vi "solar_msg Q DeQ.vi"(8 "error in (no error)":errorcluster, 9 "Timeout ms (-1)":i32=-1, 10 "CMD Timeout (\"\")":cluster{"MSG":string, "DATA":variant}, 11 "Queue in":refnum<queue>) -> (0 "error out":errorcluster, 1 "CMD_DATA":variant, 2 "CMD":string, 3 "Queue out":refnum<queue>, 4 "Timed Out?":bool)   [LabVIEW 2018]
doc: "This removes a message from the front of the queue. If timed out this returns the <b>CMD Timeout</b> message. If an error occurs this returns an 'ERROR' message. If the queue is invalid this returns an 'EXIT' message."
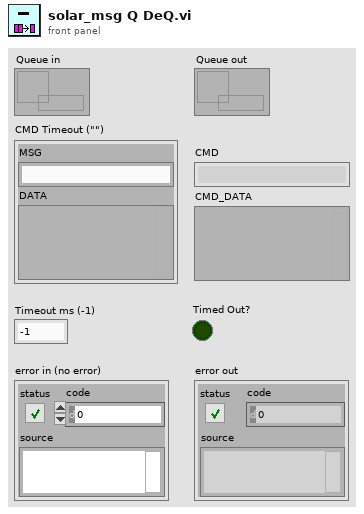
[diagram p1: front panel]
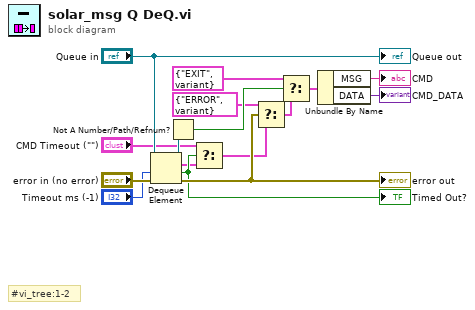
[diagram p0: block diagram]
diagram:
  # "#vi_tree:1-2"
  n1 = Dequeue Element(queue="Queue in", timeout in ms (-1)="Timeout ms (-1)", error in (no error)="error in (no error)") -> (queue out=w14:refnum<queue>, element=w8:cluster{"MSG":string, "DATA":variant}, timed out?=w9:bool, error out=w10:errorcluster)
  "error out" <- w10
  "Timed Out?" <- w9
  n2 = Not A Number/Path/Refnum?(number/path/refnum=w14) -> (NaN/Path/Refnum?=w12:bool)
  n3 = Select(t="CMD Timeout (\"\")", s=w9, f=w8) -> (s? t:f=w5:cluster{"MSG":string, "DATA":variant})
  n4 = Select(t=cluster{"MSG":string, "DATA":variant} {"MSG"="ERROR", "DATA"=variant} ("CMD Timeout (\"\")"), s=w10, f=w5) -> (s? t:f=w11:cluster{"MSG":string, "DATA":variant})
  n5 = Select(t=cluster{"MSG":string, "DATA":variant} {"MSG"="EXIT", "DATA"=variant} ("CMD Timeout (\"\")"), s=w12, f=w11) -> (s? t:f=w3:cluster{"MSG":string, "DATA":variant})
  n6 = Unbundle By Name(w3) -> ("MSG"=→"CMD":string, "DATA"=→"CMD_DATA":variant)
  "Queue out" <- "Queue in"
